vi "search same item.vi"(9 "item":string, 11 "Item Data":string[][](array[string])=[["0", "2017/2/3 20:41:53", "语义", "1", "1", "1", "1", "1", "1", "1", "1", "1"], ["1", "2017/2/3 20:43:36", "语义", "1", "1", "1", "1", "1", "1", "1", "1", "1"], ["2", "2017/2/3 20:51:23", "语义", "1", "1", "1", "1", "1", "1", "1", "1", "1"], ["3", "2017/2/3 20:51:25", "语义", "1", "1", "1", "1", "1", "1", "1", "1", "1"], ["4", "2017/2/3 20:51:26", "语义", "1", "1", "1", "1", "1", "1", "1", "1", "1"], ["5", "2017/2/3 20:51:27", "语义", "1", "1", "1", "1", "1", "1", "1", "1", "1"], ["6", "2017/2/3 20:51:29", "语义", "1", "1", "1", "1", "1", "1", "1", "1", "1"]]) -> (1 "Item ID":i32[](array[numeric]), 3 "Item Data输出":string[](array[string]))   [LabVIEW 2016]
panel:
  out "子数组":string[](array[string])
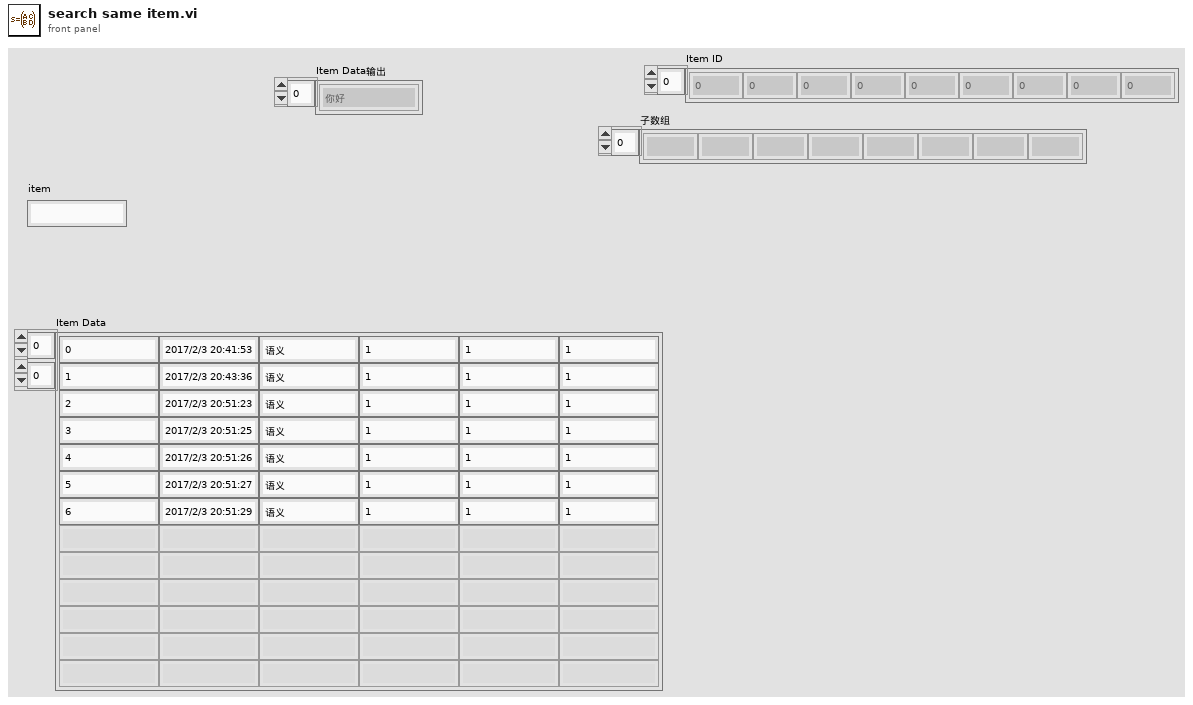
[diagram p1: front panel]
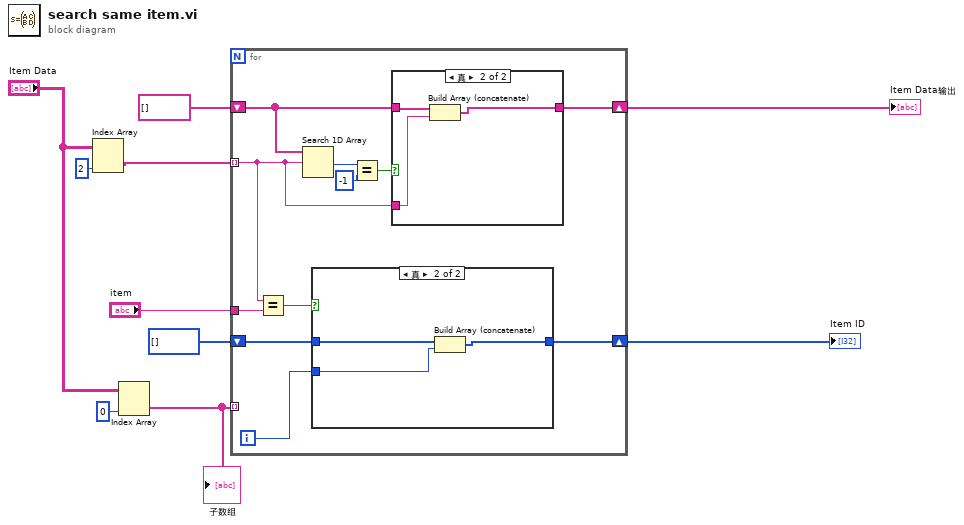
[diagram p0: block diagram]
diagram:
  n1 = Index Array(array="Item Data", index (col)=2 ("禁用的索引 (列)")) -> (element=w6:string[])  [unwired: 1 in]
  n2 = Index Array(array="Item Data", index (col)=0 ("禁用的索引 (列)")) -> (element=w3:string[])  [unwired: 1 in]
  "子数组" <- w3
  n3 = for {
    tunnel: w6 -> [w16] mode=indexing
    shift-right: [w17] -> w10
    shift-left: string[] [] ("Item Data") -> [w18]
    tunnel: "item" -> [w15]
    tunnel: w3 -> [_] mode=indexing
    shift-right: [w12] -> w1
    shift-left: i32[] [] ("Item Data") -> [w13]
    i -> [w11]
    n4 = Equal?(x=w16, y=w15) -> (x = y?=w14:bool)
    n5 = Search 1D Array(1D array=w18, element=w16) -> (index of element=w21:i32)  [unwired: 1 in]
    n6 = case shown="真" w14 {
      tunnel: [w22 w24] -> w12
      tunnel: w13 -> [w22 w25]
      tunnel: w11 -> [_ w23]
      frame False {
      }
      frame True {
        n7 = Build Array (concatenate)(w25, w23) -> (w24:i32[])
      }
    }
    n8 = Equal?(x=w21, y=-1) -> (x = y?=w19:bool)
    n9 = case shown="真" w19 {
      tunnel: w18 -> [w26 w29]
      tunnel: w16 -> [_ w28]
      tunnel: [w26 w27] -> w17
      frame False {
      }
      frame True {
        n10 = Build Array (concatenate)(w29, w28) -> (w27:string[])
      }
    }
  }
  "Item Data输出" <- w10
  "Item ID" <- w1
